vi "LvMPDC_CMD_status.vi"(6 "timeout_ms":i32=25000, 8 "error in (no error)":errorcluster, 9 "ReadBytes":i32=1024, 11 "Connect ID":refnum<k5>) -> (0 "error out":errorcluster, 1 "status":T1 {"elapsed" format="%<%H:%M:%S%3u>t"; "time" format="%<%H:%M:%S%3u>t"}, 3 "Connect ID out":refnum<k5>)   [LabVIEW 2012]
uses:
  LvMPDC_Typdef_status.ctl
panel:
  # "status(playing) reply:\n\"OK MPD 0.16.0\nvolume: 90\nrepeat: 0\nrandom: 0\nsingle: 0\nconsume: 1\nplaylist: 10\nplaylistlength: 6\nxfade: 0\nmixrampdb: 0.000000\nmixrampdelay: nan\nstate: play\nsong: 0\nsongid: 8\ntime: 48:264\nelapsed: 47.833\nbitrate: 128\naudio: 22050:24:1\nnextsong: 1\nnextsongid: 9\nOK\n\"\n\n\nstatus(idle) reply: \n\"OK MPD 0.16.0\nvolume: 90\nrepeat: 0\nrandom: 0\nsingle: 0\nconsume: 1\nplaylist: 16\nplaylistlength: 0\nxfade: 0\nmixrampdb: 0.000000\nmixrampdelay: nan\nstate: stop\nOK\n\""
  # "LvMPDC:: CMD status"
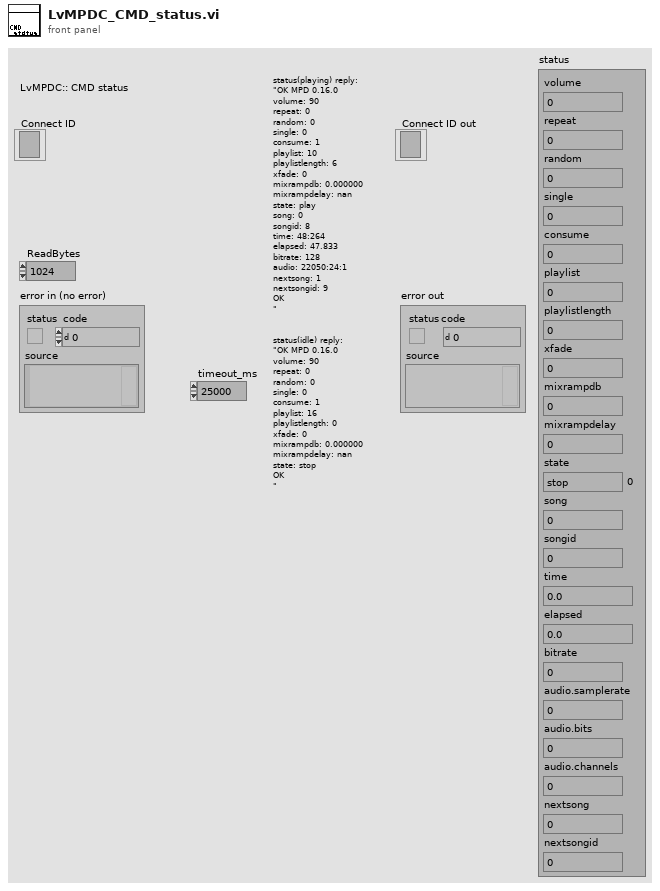
[diagram p1: front panel]
types:
  T1 = typedef "LvMPDC_Typdef_status.ctl" = cluster{"volume":i32, "repeat":i32, "random":i32, "single":i32, "consume":i32, "playlist":i32, "playlistlength":i32, "xfade":i32, "mixrampdb":dbl, "mixrampdelay":dbl, "state":enum16{"stop", "play", "pause"}, "song":i32, "songid":i32, "time":dbl, "elapsed":dbl, "bitrate":i32, "audio.samplerate":i32, "audio.bits":i32, "audio.channels":i32, "nextsong":i32, "nextsongid":i32}
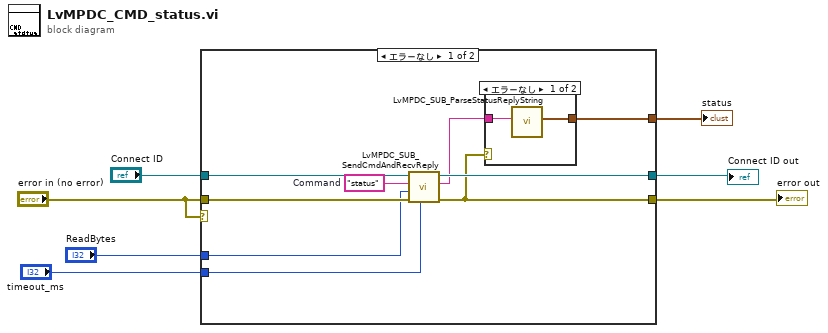
[diagram p0: block diagram]
diagram:
  n1 = case shown="エラーなし" "error in (no error)" {
    tunnel: "Connect ID" -> [w15 w20]
    tunnel: "error in (no error)" -> [w16 w19]
    tunnel: [w14 w20] -> w6
    tunnel: [w10 w19] -> w5
    tunnel: "timeout_ms" -> [w11 _]
    tunnel: "ReadBytes" -> [w12 _]
    tunnel: [w8 _] -> w1
    frame No Error {
      w13 = "status"  # Command
      n2 = call "LvMPDC_SUB_SendCmdAndRecvReply.vi"("timeout_ms"=w11, "error in (no error)"=w16, "ReadBytes"=w12, "Command"=w13, "Connect ID"=w15) -> ("error out"=w10:errorcluster, "Reply"=w9:string, "Connect ID out"=w14:refnum<k5>)  [unwired: 4 in]
      n3 = case shown="エラーなし" w10 {
        tunnel: w9 -> [w18 _]
        tunnel: [w17 _] -> w8
        frame No Error {
          n4 = call "LvMPDC_SUB_ParseStatusReplyString.vi"("status reply string"=w18) -> ("status"=w17:T1)  [unwired: 10 in]
        }
        frame Error {
        }
      }
    }
    frame Error {
    }
  }
  "Connect ID out" <- w6
  "error out" <- w5
  "status" <- w1
